vi "Calibration File Parse.vi"(7 "Calibration Coefficients":dbl[][](array[numeric]), 8 "34972 Array":dbl[](array[numeric]), 9 "MW100 Array":dbl[](array[numeric])) -> (2 "34972 Calibration":dbl[](array[numeric]) format="%_4g", 3 "MW100 Calibration":dbl[](array[numeric]))   [LabVIEW 2012]
doc: "This VI parses a calibration file located a C:\\work and applies the correction coefficient to both the 34972 and MW100 arrays"
panel:
  out "MW Coefficients":dbl[](array[numeric])
  out "34792 Coefficients":dbl[](array[numeric])
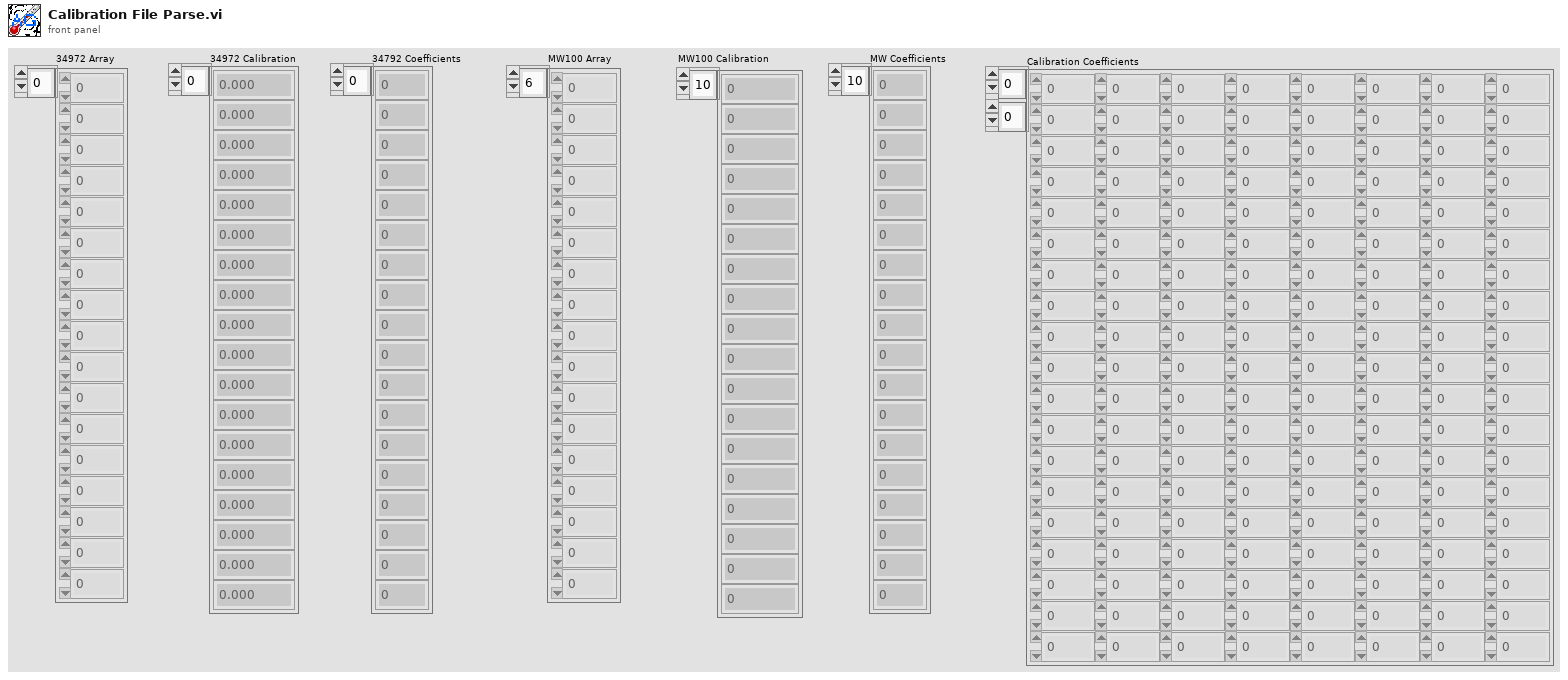
[diagram p1: front panel]
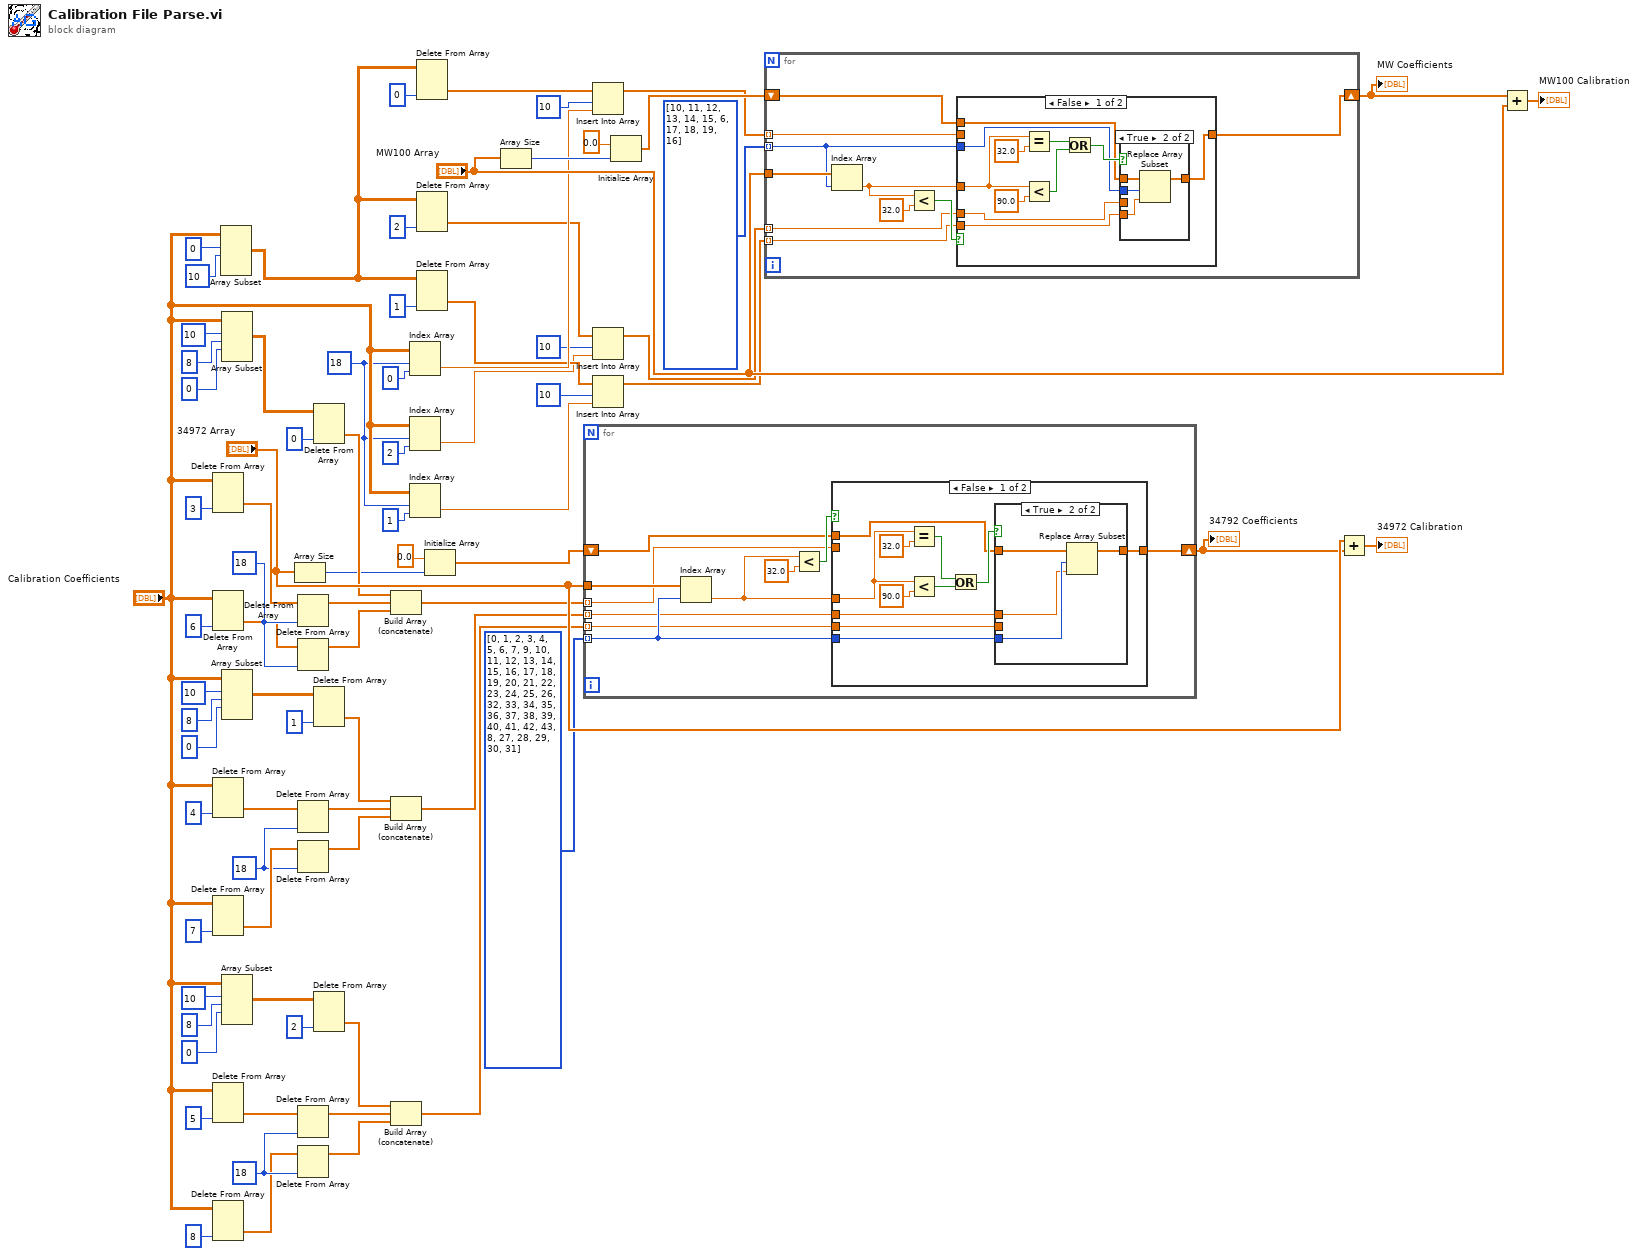
[diagram p0: block diagram]
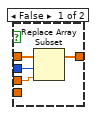
[diagram p2: hidden frame]
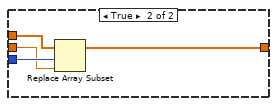
[diagram p3: hidden frame]
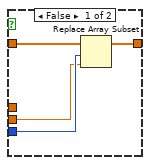
[diagram p4: hidden frame]
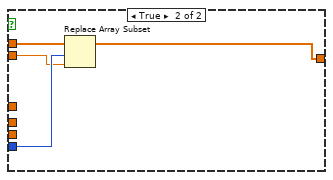
[diagram p5: hidden frame]
diagram:
  w11 = 18 ("disabled index (row)")
  w42 = 18 ("index (row)")
  w59 = 18 ("index (row)")
  w67 = 18 ("index (row)")
  n1 = Delete From Array(array="Calibration Coefficients", index (col)=3 ("disabled index (col)")) -> (deleted portion=w66:dbl[])  [unwired: 2 in, 1 out]
  n2 = Delete From Array(array="Calibration Coefficients", index (col)=6 ("disabled index (col)")) -> (deleted portion=w65:dbl[])  [unwired: 2 in, 1 out]
  n3 = Delete From Array(array="Calibration Coefficients", index (col)=4 ("disabled index (col)")) -> (deleted portion=w60:dbl[])  [unwired: 2 in, 1 out]
  n4 = Delete From Array(array="Calibration Coefficients", index (col)=7 ("disabled index (col)")) -> (deleted portion=w61:dbl[])  [unwired: 2 in, 1 out]
  n5 = Delete From Array(array="Calibration Coefficients", index (col)=5 ("disabled index (col)")) -> (deleted portion=w41:dbl[])  [unwired: 2 in, 1 out]
  n6 = Delete From Array(array="Calibration Coefficients", index (col)=8 ("disabled index (col)")) -> (deleted portion=w40:dbl[])  [unwired: 2 in, 1 out]
  n7 = Array Subset(array="Calibration Coefficients", index (row)=0 ("index"), length (row)=10 ("length")) -> (w28:dbl[][])  [unwired: 2 in]
  n8 = Array Subset(array="Calibration Coefficients", index (row)=10 ("index"), length (row)=8 ("length"), index (col)=0 ("index")) -> (w1:dbl[][])  [unwired: 1 in]
  n9 = Array Subset(array="Calibration Coefficients", index (row)=10 ("index"), length (row)=8 ("length"), index (col)=0 ("index")) -> (w54:dbl[][])  [unwired: 1 in]
  n10 = Array Subset(array="Calibration Coefficients", index (row)=10 ("index"), length (row)=8 ("length"), index (col)=0 ("index")) -> (w47:dbl[][])  [unwired: 1 in]
  n11 = Array Size(array="34972 Array") -> (size(s)=w36:i32)
  n12 = Delete From Array(array=w66, index=w67) -> (array with subset deleted=w64:dbl[])  [unwired: 1 in, 1 out]
  n13 = Delete From Array(array=w65, index=w67) -> (array with subset deleted=w63:dbl[])  [unwired: 1 in, 1 out]
  n14 = Delete From Array(array=w60, index=w59) -> (array with subset deleted=w62:dbl[])  [unwired: 1 in, 1 out]
  n15 = Delete From Array(array=w61, index=w59) -> (array with subset deleted=w3:dbl[])  [unwired: 1 in, 1 out]
  n16 = Delete From Array(array=w41, index=w42) -> (array with subset deleted=w39:dbl[])  [unwired: 1 in, 1 out]
  n17 = Delete From Array(array=w40, index=w42) -> (array with subset deleted=w38:dbl[])  [unwired: 1 in, 1 out]
  n18 = Delete From Array(array=w1, index (col)=0 ("disabled index (col)")) -> (deleted portion=w68:dbl[])  [unwired: 2 in, 1 out]
  n19 = Delete From Array(array=w54, index (col)=1 ("disabled index (col)")) -> (deleted portion=w58:dbl[])  [unwired: 2 in, 1 out]
  n20 = Delete From Array(array=w47, index (col)=2 ("disabled index (col)")) -> (deleted portion=w43:dbl[])  [unwired: 2 in, 1 out]
  n21 = Build Array (concatenate)(w68, w64, w63) -> (w32:dbl[])
  n22 = Build Array (concatenate)(w58, w62, w3) -> (w2:dbl[])
  n23 = Build Array (concatenate)(w43, w39, w38) -> (w33:dbl[])
  n24 = Index Array(array="Calibration Coefficients", index (row)=w11, index (col)=0 ("disabled index (row)")) -> (element=w16:dbl)
  n25 = Index Array(array="Calibration Coefficients", index (row)=w11, index (col)=2 ("disabled index (row)")) -> (element=w10:dbl)
  n26 = Index Array(array="Calibration Coefficients", index (row)=w11, index (col)=1 ("disabled index (row)")) -> (element=w13:dbl)
  n27 = Delete From Array(array=w28, index (col)=0 ("disabled index (col)")) -> (deleted portion=w17:dbl[])  [unwired: 2 in, 1 out]
  n28 = Delete From Array(array=w28, index (col)=2 ("disabled index (col)")) -> (deleted portion=w9:dbl[])  [unwired: 2 in, 1 out]
  n29 = Delete From Array(array=w28, index (col)=1 ("disabled index (col)")) -> (deleted portion=w12:dbl[])  [unwired: 2 in, 1 out]
  n30 = Initialize Array(0.0 ("element"), w36) -> (w34:dbl[])
  n31 = Array Size(array="MW100 Array") -> (size(s)=w23:i32)
  n32 = for {
    tunnel: i32[] [0, 1, 2, 3, 4, 5, 6, 7, 9, 10, 11, 12, 13, 14, 15, 16, 17, 18, 19, 20, 21, 22, 23, 24, 25, 26, 32, 33, 34, 35, 36, 37, 38, 39, 40, 41, 42, 43, 8, 27, 28, 29, 30, 31] -> [w84] mode=indexing
    tunnel: "34972 Array" -> [w89]
    tunnel: w32 -> [w83] mode=indexing
    shift-right: [w85] -> w31
    shift-left: w34 -> [w86]
    tunnel: w2 -> [w82] mode=indexing
    tunnel: w33 -> [w81] mode=indexing
    n33 = Index Array(array=w89, index=w84) -> (element=w80:dbl)
    n34 = Less?(x=w80, y=32.0) -> (x < y?=w87:bool)
    n35 = case shown="False" w87 {
      tunnel: w83 -> [_ w109]
      tunnel: w80 -> [w93 _]
      tunnel: w86 -> [w95 w112]
      tunnel: w84 -> [w94 w111]
      tunnel: [w91 w110] -> w85
      tunnel: w82 -> [w92 _]
      tunnel: w81 -> [w90 _]
      frame False {
        n36 = Equal?(x=w93, y=32.0) -> (x = y?=w99:bool)
        n37 = Less?(x=w93, y=90.0) -> (x < y?=w97:bool)
        n38 = Or(x=w99, y=w97) -> (x .or. y?=w96:bool)
        n39 = case shown="True" w96 {
          tunnel: w95 -> [w104 w108]
          tunnel: w94 -> [w102 w107]
          tunnel: w92 -> [_ w105]
          tunnel: [w103 w106] -> w91
          tunnel: w90 -> [w101 _]
          frame False {
            n40 = Replace Array Subset(array=w104, new element=w101, index=w102) -> (w103:dbl[])
          }
          frame True {
            n41 = Replace Array Subset(array=w108, new element=w105, index=w107) -> (w106:dbl[])
          }
        }
      }
      frame True {
        n42 = Replace Array Subset(array=w112, new element=w109, index=w111) -> (w110:dbl[])
      }
    }
  }
  "34792 Coefficients" <- w31
  n43 = Insert Into Array(array=w17, index=10, new element=w16) -> (w15:dbl[])
  n44 = Insert Into Array(array=w9, index=10, new element=w10) -> (w8:dbl[])
  n45 = Insert Into Array(array=w12, index=10, new element=w13) -> (w14:dbl[])
  n46 = Initialize Array(0.0 ("element"), w23) -> (w21:dbl[])
  n47 = for {
    tunnel: i32[] [10, 11, 12, 13, 14, 15, 6, 17, 18, 19, 16] -> [w117] mode=indexing
    tunnel: "MW100 Array" -> [w122]
    tunnel: w15 -> [w116] mode=indexing
    shift-right: [w118] -> w24
    shift-left: w21 -> [w119]
    tunnel: w14 -> [w115] mode=indexing
    tunnel: w8 -> [w114] mode=indexing
    n48 = Index Array(array=w122, index=w117) -> (element=w113:dbl)
    n49 = Less?(x=w113, y=32.0) -> (x < y?=w120:bool)
    n50 = case shown="False" w120 {
      tunnel: w116 -> [_ w142]
      tunnel: w113 -> [w126 _]
      tunnel: w119 -> [w128 w145]
      tunnel: w117 -> [w127 w144]
      tunnel: [w124 w143] -> w118
      tunnel: w115 -> [w125 _]
      tunnel: w114 -> [w123 _]
      frame False {
        n51 = Equal?(x=w126, y=32.0) -> (x = y?=w132:bool)
        n52 = Less?(x=w126, y=90.0) -> (x < y?=w130:bool)
        n53 = Or(x=w132, y=w130) -> (x .or. y?=w129:bool)
        n54 = case shown="True" w129 {
          tunnel: w128 -> [w137 w141]
          tunnel: w127 -> [w135 w140]
          tunnel: w125 -> [_ w138]
          tunnel: [w136 w139] -> w124
          tunnel: w123 -> [w134 _]
          frame False {
            n55 = Replace Array Subset(array=w137, new element=w134, index=w135) -> (w136:dbl[])
          }
          frame True {
            n56 = Replace Array Subset(array=w141, new element=w138, index=w140) -> (w139:dbl[])
          }
        }
      }
      frame True {
        n57 = Replace Array Subset(array=w145, new element=w142, index=w144) -> (w143:dbl[])
      }
    }
  }
  "MW Coefficients" <- w24
  n58 = Add(x="34972 Array", y=w31) -> (x+y=→"34972 Calibration":dbl[])
  n59 = Add(x=w24, y="MW100 Array") -> (x+y=→"MW100 Calibration":dbl[])
